vi "Save Settings To File.vi"(8 "error in":errorcluster, 10 "Drive PID":T1, 11 "refnum":T2) -> (0 "error out":errorcluster, 3 "refnum out":T2)   [LabVIEW 2016]
uses:
  <vilib>/Utility/config.llb/Config Data RefNum.ctl
  PID Settings.ctl
  <vilib>/Utility/config.llb/NI_LVConfig.lvlib
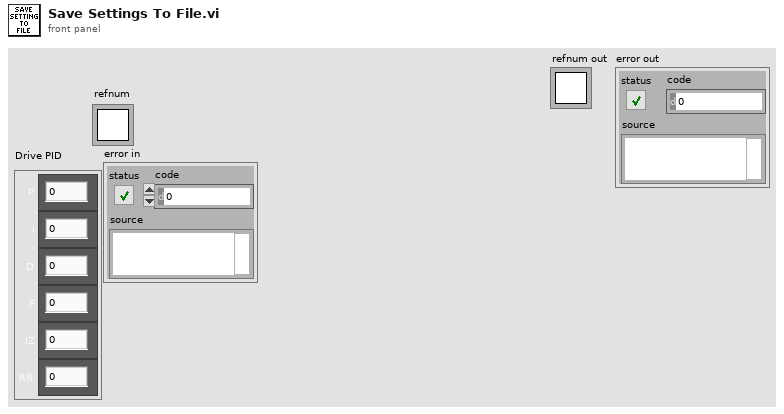
[diagram p1: front panel]
types:
  T1 = typedef "PID Settings.ctl" = cluster{"D":dbl, "F":dbl, "RR":dbl, "IZ":dbl, "P":dbl, "I":dbl}
  T2 = typedef "NI_LVConfig.lvlib/Config Data RefNum.ctl" = refnum<k1>
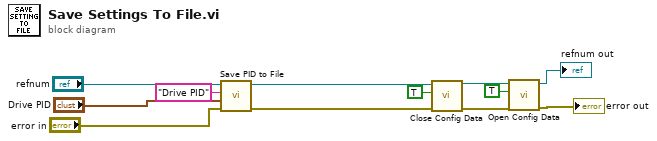
[diagram p0: block diagram]
diagram:
  n1 = call "Save PID to File.vi"("error in"="error in", "PID"="Drive PID", "Name"="Drive PID", "refnum in"="refnum") -> ("error out"=w2:errorcluster, "refnum out"=w8:T2)  [unwired: 6 in]
  n2 = call <vilib>:"Close Config Data.vi"("error in (no error)"=w2, "write file if changed (T)"=TRUE, "refnum"=w8) -> ("error out"=w5:errorcluster, "file path"=w7:path)  [unwired: 7 in]
  n3 = call <vilib>:"Open Config Data.vi"("error in (no error)"=w5, "create file if necessary (T)"=TRUE, "configuration file path"=w7) -> ("error out"=→"error out":errorcluster, "refnum"=→"refnum out":T2)  [unwired: 6 in, 1 out]
